vi "Initialize Attributes.vi"(8 "error in (no error)":errorcluster, 10 "Attribute Data":variant, 11 "CS++BaseActor in":refnum<class "CS++BaseActor.lvclass">) -> (0 "error out":errorcluster, 2 "Found?":bool, 3 "CS++BaseActor out":refnum<class "CS++BaseActor.lvclass">)   [LabVIEW 2012, in "CS++BaseActor.lvlib" / "CS++BaseActor.lvclass"]
doc: "Initialize object attribute.\n\nUnique resources should be allocated elsewhere!"
uses:
  CS++BaseActor.lvclass
  CS++BaseActor.lvclass/CS++BaseActor.ctl
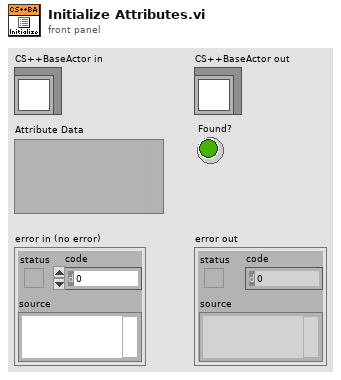
[diagram p1: front panel]
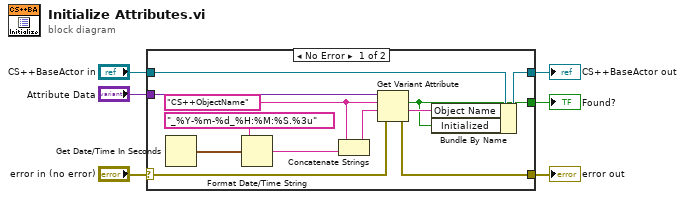
[diagram p0: block diagram]
diagram:
  n1 = case shown="No Error" "error in (no error)" {
    selector: "error in (no error)" -> [w12 w20]
    tunnel: [w11 w20] -> w1
    tunnel: [w17 w19] -> w5
    tunnel: "CS++BaseActor in" -> [w18 w19]
    tunnel: "Attribute Data" -> [w16 _]
    tunnel: [w7 _] -> w3
    frame No Error {
      w9 = "CS++ObjectName" ("name")
      n2 = Get Date/Time In Seconds() -> (seconds since 1Jan1904=w15:timestamp)
      n3 = Format Date/Time String(time format string (%c)="_%Y-%m-%d_%H:%M:%S.%3u", seconds (now)=w15) -> (date/time string=w13:string)  [unwired: 1 in]
      n4 = Concatenate Strings(w9, w13) -> (w10:string)
      n5 = Get Variant Attribute(Variant=w16, name=w9, default value (empty Variant)=w10, error in=w12) -> (found=w7:bool, value=w8:string, error out=w11:errorcluster)  [unwired: 1 out]
      n6 = Bundle By Name(cluster=w18, "Object Name"=w8, "Initialized"=w7) -> (w17:refnum<class "CS++BaseActor.lvclass">)
    }
    frame Error {
    }
  }
  "error out" <- w1
  "CS++BaseActor out" <- w5
  "Found?" <- w3
